vi "Memory.Pointer.Block Descriptor to Object.vi"(8 "error in (no error)":errorcluster, 10 "block descriptor":cluster{"address":u64, "size":u64} {"address" format="%016x"; "size" format="%d bytes"}, 11 "pointer in":refnum<class "Memory.Pointer.lvclass">) -> (0 "error out":errorcluster, 3 "pointer out":refnum<class "Memory.Pointer.lvclass">)   [LabVIEW 2016, in "Memory Manager.lvlib" / "Memory.Pointer.lvclass"]
uses:
  Memory.Pointer.lvclass
  Memory.Pointer.lvclass/Memory.Pointer.ctl
  Memory.Pointer.Errors.vi
  Memory.Pointer.Errors.Null Pointer.vi
  Accessors/Get Address.vi
  Memory.Pointer.Errors.Create Error.vi
  Submodules/SEH/Source/VIs/Static Error Handling.Error Cluster Constant.vi
  Submodules/SEH/Source/VIs/Static Error Handling.Error Cluster Constant (256B).vi
  Submodules/SEH/Source/VIs/Static Error Handling.Parameters.Status.Set.vi
  Submodules/SEH/Source/VIs/Static Error Handling.Parameters.Code.Set.vi
  Submodules/SEH/Source/VIs/Static Error Handling.Parameters.VI Source.Set.vi
  Constants/Memory.Constants.vi
  Constants/Memory.Constants.Library Name.vi
  Memory.Pointer.Errors.Get Info.vi
  Submodules/SEH/Source/VIs/Static Error Handling.Source Buffer.Write.String.vi
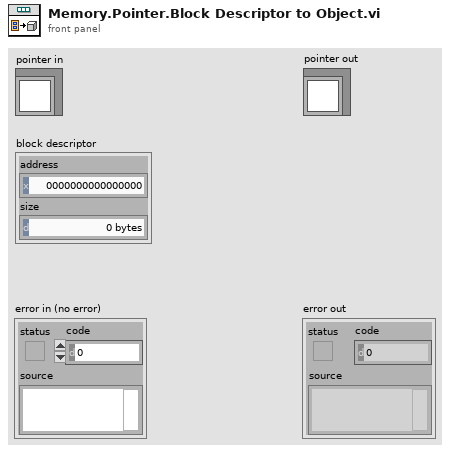
[diagram p1: front panel]
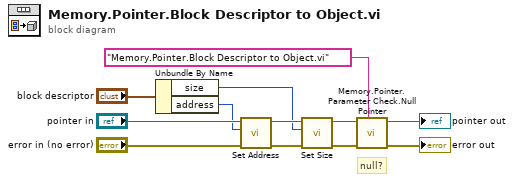
[diagram p0: block diagram]
diagram:
  # "null?"
  n1 = Unbundle By Name("block descriptor") -> ("size"=w6:u64, "address"=w7:u64)
  n2 = call "Set Address.vi"("error in (no error)"="error in (no error)", "address"=w7, "Pointer in"="pointer in") -> ("error out"=w11:errorcluster, "Pointer out"=w8:refnum<class "Memory.Pointer.lvclass">)  [unwired: 7 in]
  n3 = call "Set Size.vi"("error in (no error)"=w11, "size"=w6, "Pointer in"=w8) -> ("error out"=w3:errorcluster, "Pointer out"=w4:refnum<class "Memory.Pointer.lvclass">)  [unwired: 7 in]
  n4 = call "Memory.Pointer.Parameter Check.Null Pointer.vi"("source vi name"="Memory.Pointer.Block Descriptor to Object.vi", "error in (no error)"=w3, "Pointer in"=w4) -> ("error out"=→"error out":errorcluster, "Pointer out"=→"pointer out":refnum<class "Memory.Pointer.lvclass">)  [unwired: 7 in]
